vi "get Data Store.vi"(11 "Actor in":refnum<class "Actor.lvclass">) -> (3 "Data Store":refnum<data-value>)   [LabVIEW 2015]
uses:
  Actor.lvclass
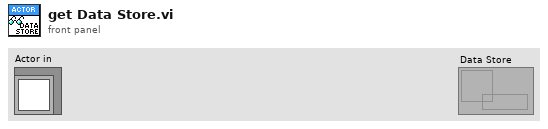
[diagram p1: front panel]
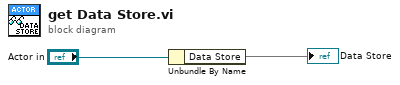
[diagram p0: block diagram]
diagram:
  n1 = Unbundle By Name("Actor in") -> ("Data Store"=→"Data Store")
